vi "Lab1Labview.vi"() -> ()   [LabVIEW 2024]
panel:
  out "Boolean":bool
  out "Flow Rate":dbl(slide) scale=-40000.0..40000.0
  out "\"SCC Volts":dbl format="%_3f"
  out "AD2 Input":i16 format="%04x"
  in  "stop":bool
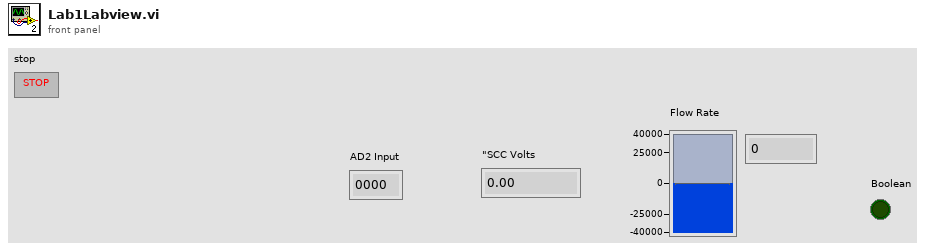
[diagram p1: front panel]
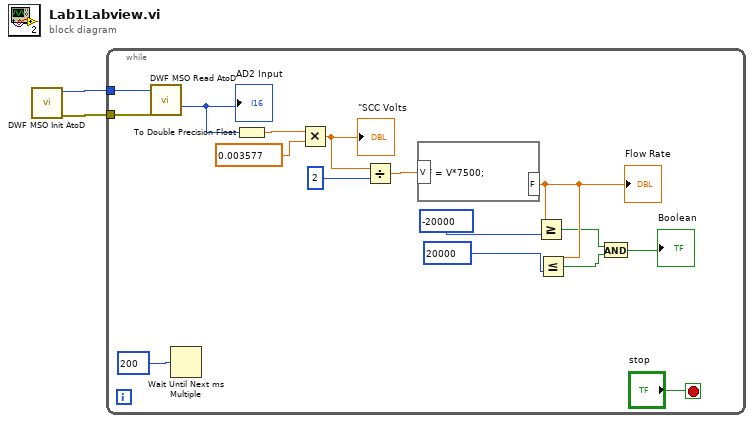
[diagram p0: block diagram]
diagram:
  n1 = call "DWF MSO Init AtoD.vi"() -> ("Error Out"=w1:errorcluster, "Instrument Handle Out"=w2:u32)  [unwired: 10 in]
  n2 = while {
    tunnel: w2 -> [w17]
    tunnel: w1 -> [w16]
    stop <- "stop" stop-if-true
    n3 = call "DWF MSO Read AtoD.vi"("Instrument Handle In AtoD"=w17, "Error In"=w16) -> ("AtoD"=w12:i16)  [unwired: 12 in, 1 out]
    "AD2 Input" <- w12
    n4 = Wait Until Next ms Multiple(millisecond multiple=200) -> ()  [unwired: 1 out]
    n5 = To Double Precision Float(number=w12) -> (double precision float=w14:dbl)
    n6 = Multiply(x=w14, y=0.003577) -> (x*y=w11:dbl)
    "\"SCC Volts" <- w11
    n7 = Divide(x=w11, y=2) -> (x/y=w9:dbl)
    n8 = formula code="F = V*7500;"("V"=w9) -> ("F"=w8:dbl)
    "Flow Rate" <- w8
    n9 = Greater Or Equal?(x=w8, y=-20000) -> (x >= y?=w4:bool)
    n10 = Less Or Equal?(x=w8, y=20000) -> (x <= y?=w5:bool)
    n11 = And(x=w4, y=w5) -> (x .and. y?=→"Boolean":bool)
  }
